vi "MathOptim-Power 2 Full Parameter Vector.vi"(0 "Y":dbl[](array[numeric]) format="%.2f", 5 "X":dbl[](array[numeric]), 7 "a":dbl[](array[numeric])) -> (8 "parameters":dbl[](array[numeric]))   [LabVIEW 2020]
doc: "This template is the starting point for creating a model function to be passed to the Nonlinear Curve Fit.vi."
uses:
  <vilib>/Analysis/7linalg.llb/Solve Linear Equations (single right hand).vi
  <vilib>/Analysis/baseanly.llb/Solve Linear Equations By Cholesky.vi
  <vilib>/Analysis/baseanly.llb/Real Matrix to Compact Array.vi
  <vilib>/Analysis/baseanly.llb/Real Compact Tri-Matrix Linear Eqs.vi
  <vilib>/Analysis/7linalg.llb/Solve Linear Eqs (General).vi
  <vilib>/Analysis/7linalg.llb/Solve Linear Eqs (Gen, single right hand).vi
  <vilib>/Analysis/NI_AALPro.lvlib
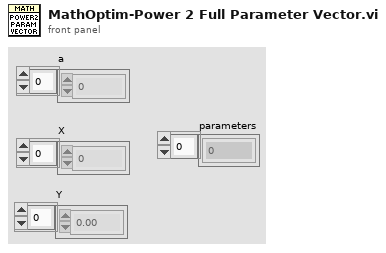
[diagram p1: front panel]
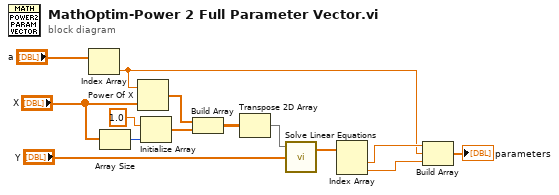
[diagram p0: block diagram]
diagram:
  n1 = Index Array(array="a") -> (element=w3:dbl)  [unwired: 1 in]
  n2 = Array Size(array="X") -> (size(s)=w13:i32)
  n3 = Power Of X(1:"X", 2:w3) -> (0:w6:dbl[])
  n4 = Initialize Array(1.0, w13) -> (w11:dbl[])
  n5 = Build Array(w6, w11) -> (w10:dbl[][])
  n6 = Transpose 2D Array(2D array=w10) -> (transposed array=w7:dbl[][])
  n7 = call-poly <vilib>:"Solve Linear Equations.vi"("Known Vector"="Y", "Input Matrix"=w7) -> ("Solution Vector"=w9:dbl[])  [unwired: 1 in, 1 out]
  n8 = Index Array(array=w9) -> (element #1=w5:dbl, element #2=w4:dbl)  [unwired: 2 in]
  n9 = Build Array(w5, w3, w4) -> (→"parameters":dbl[])
